vi "Save_data.vi"(0 "Data to be saved":dbl[][](array[numeric]), 1 "Save tiff stack?":bool, 5 "File name":string, 7 "Save?":bool, 9 "Append?":bool=TRUE, 11 "error in (no error)":errorcluster) -> (4 "Appended path":path, 15 "error out":errorcluster)   [LabVIEW 2014]
uses:
  <vilib>/Utility/file.llb/Write To Spreadsheet File (DBL).vi
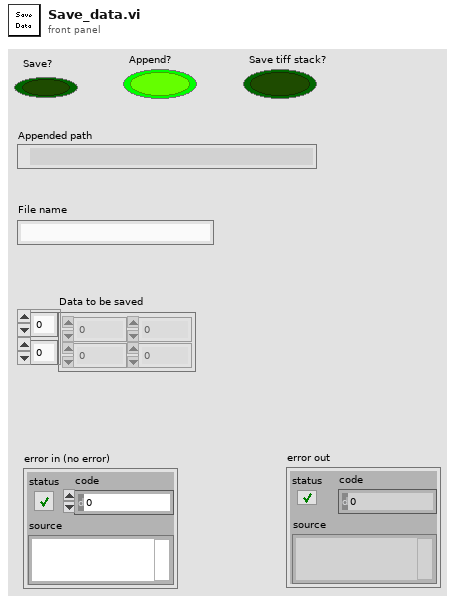
[diagram p1: front panel]
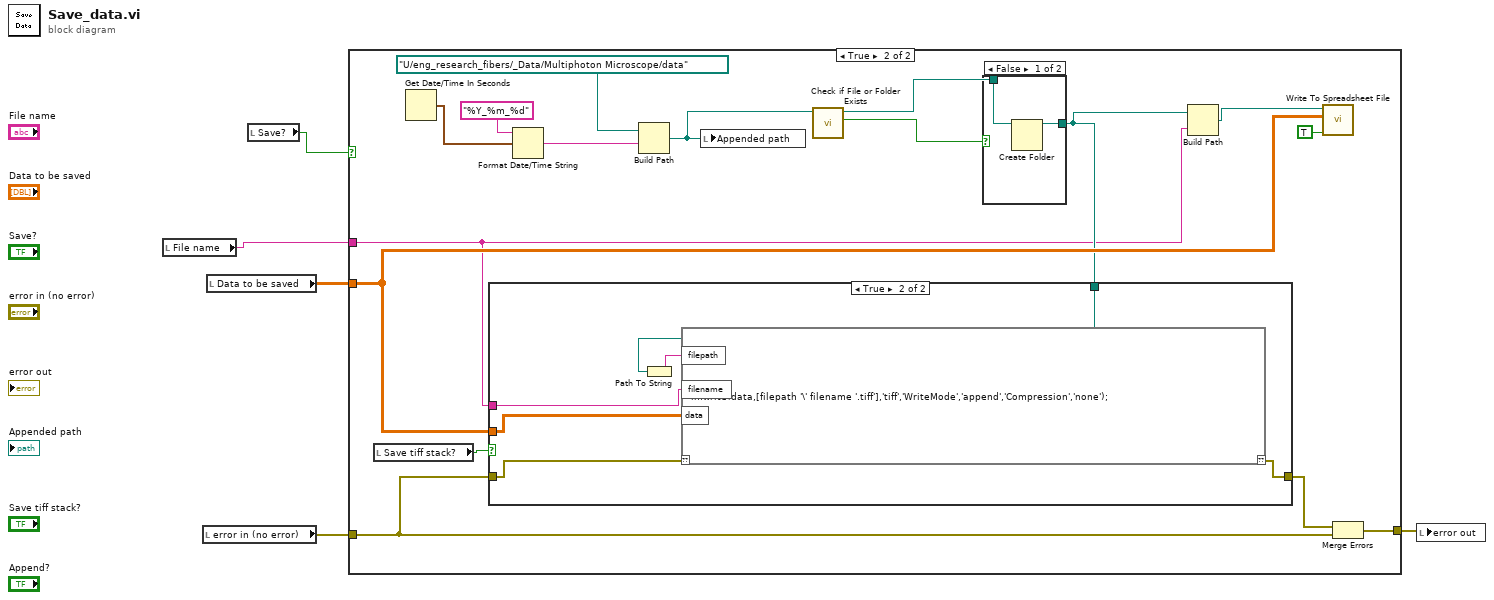
[diagram p0: block diagram]
diagram:
  n1 = local read "File name"() -> (w1:string)
  n2 = local read "error in (no error)"() -> (w3:errorcluster)
  n3 = local read "Data to be saved"() -> (w4:dbl[][])
  n4 = local read "Save?"() -> (w5:bool)
  n5 = case shown="True" w5 {
    tunnel: w1 -> [_ w7]
    tunnel: w4 -> [_ w13]
    tunnel: w3 -> [w6 w17]
    tunnel: [w6 w15] -> w2
    frame False {
    }
    frame True {
      n6 = local read "Save tiff stack?"() -> (w14:bool)
      n7 = Get Date/Time In Seconds() -> (seconds since 1Jan1904=w8:timestamp)
      n8 = Format Date/Time String(time format string (%c)="%Y_%m_%d", seconds (now)=w8) -> (date/time string=w9:string)  [unwired: 1 in]
      n9 = Build Path(base path=path "U:/eng_research_fibers/_Data/Multiphoton Microscope/data", name or relative path=w9) -> (appended path=w18:path)
      n10 = local write "Appended path"(w18) -> ()
      n11 = call <vilib>:"Check if File or Folder Exists.vi"("path"=w18) -> ("file or folder exists?"=w21:bool, "dup path"=w20:path)  [unwired: 8 in, 1 out]
      n12 = case shown="False" w21 {
        tunnel: [w31 w32] -> w12
        tunnel: w20 -> [w30 w32]
        frame False {
          n13 = Create Folder(path (use dialog)=w30) -> (created path=w31:path)  [unwired: 2 in, 2 out]
        }
        frame True {
        }
      }
      n14 = case shown="True" w14 {
        tunnel: w17 -> [w23 w29]
        tunnel: [w23 w28] -> w16
        tunnel: w13 -> [_ w27]
        tunnel: w12 -> [_ w26]
        tunnel: w7 -> [_ w24]
        frame False {
        }
        frame True {
          n15 = Path To String(path=w26) -> (string=w25:string)
          n16 = script code="imwrite(data,[filepath '\\' filename '.tiff'],'tiff','WriteMode','append','Compression','none');"("??"=w29, "data"=w27, "filepath"=w25, "filename"=w24) -> ("??"=w28:errorcluster)
        }
      }
      n17 = Build Path(base path=w12, name or relative path=w7) -> (appended path=w10:path)
      n18 = call-poly <vilib>:"Write To Spreadsheet File.vi"("append to file? (new file:F)"=TRUE, "2D data"=w13, "file path (dialog if empty)"=w10) -> ()  [unwired: 5 in, 1 out]
      n19 = Merge Errors(w16, w17) -> (w15:errorcluster)
    }
  }
  n20 = local write "error out"(w2) -> ()
